vi "eventILCCommunication.vi"(8 "error in (no error)":errorcluster, 9 "TimeoutActuatorIds":i32[](array[numeric]), 10 "Timestamp":T1, 11 "Publisher in":refnum<class "Publisher.lvclass">) -> (0 "error out":errorcluster, 3 "Publisher out":refnum<class "Publisher.lvclass">)   [LabVIEW 2016, in "Publisher.lvclass"]
uses:
  Publisher.lvclass
  DataTypes/Topics/Parts/Timestamp.ctl
  Publisher.lvclass/Publisher.ctl
  DataTypes/Topics/EventILCCommunication.ctl
  Communicator/M1M3SAL/M1M3SAL.lvclass/M1M3SAL.ctl
  Communicator/M1M3SAL/writeHeader.vi
  Communicator/M1M3SAL/writeDBL.vi
  Communicator/M1M3SAL/writeI32.vi
  Communicator/M1M3SAL/writeBoolean.vi
  Communicator/M1M3SAL/writeU8.vi
  DataTypes/Topics/M1M3SupportTopics.lvlib
  Communicator/M1M3SAL/M1M3SAL.lvclass
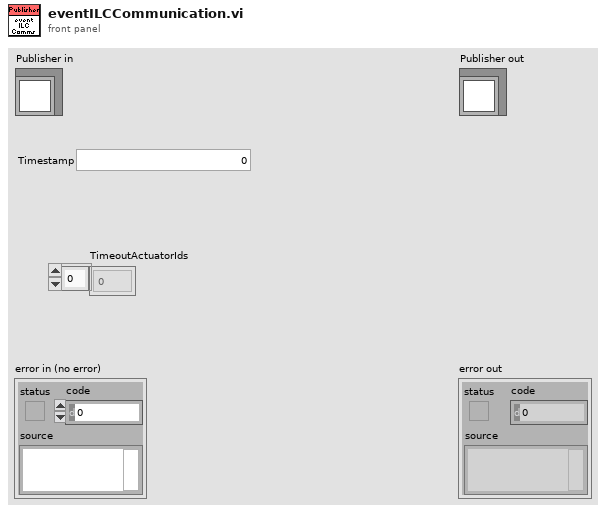
[diagram p1: front panel]
types:
  T1 = typedef "M1M3SupportTopics.lvlib/Timestamp.ctl" = dbl
  T2 = typedef "M1M3SupportTopics.lvlib/EventILCCommunication.ctl" = cluster{"Timestamp":T1, "ActuatorId":i32, "CommunicationOK":bool}
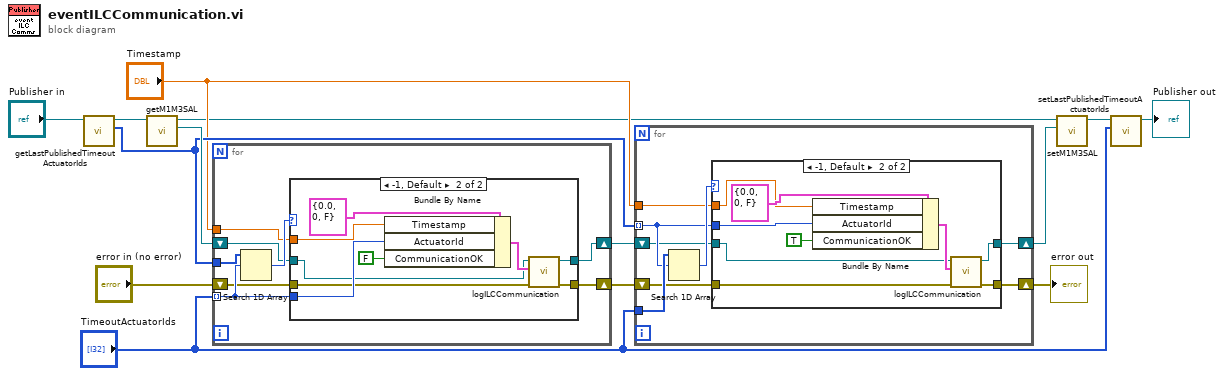
[diagram p0: block diagram]
diagram:
  n1 = call "getLastPublishedTimeoutActuatorIds.vi"("Publisher in"="Publisher in") -> ("LastPublishedTimeoutActuatorIds"=w11:i32[], "Publisher out"=w13:refnum<class "Publisher.lvclass">)  [unwired: 9 in]
  n2 = call "getM1M3SAL.vi"("Publisher in"=w13) -> ("M1M3SAL"=w12:refnum<class "M1M3SAL.lvclass">, "Publisher out"=w6:refnum<class "Publisher.lvclass">)  [unwired: 9 in]
  n3 = for {
    tunnel: "TimeoutActuatorIds" -> [w20] mode=indexing
    tunnel: w11 -> [w22]
    tunnel: "Timestamp" -> [w19]
    shift-right: [w17] -> w1
    shift-left: w12 -> [w18]
    shift-right: [w15] -> w3
    shift-left: "error in (no error)" -> [w16]
    n4 = Search 1D Array(1D array=w22, element=w20) -> (index of element=w21:i32)  [unwired: 1 in]
    n5 = case shown="-1, Default" w21 {
      tunnel: w20 -> [_ w31]
      tunnel: w19 -> [_ w30]
      tunnel: w18 -> [w24 w28]
      tunnel: [w24 w27] -> w17
      tunnel: w16 -> [w23 w26]
      tunnel: [w23 w25] -> w15
      frame 0 {
      }
      frame -1, Default {
        n6 = Bundle By Name(cluster=T2 {"Timestamp"=0.0, "ActuatorId"=0, "CommunicationOK"=FALSE} ("EventILCCommunication"), "Timestamp"=w30, "ActuatorId"=w31, "CommunicationOK"=FALSE) -> (w29:T2)
        n7 = call "logILCCommunication.vi"("error in (no error)"=w26, "EventILCCommunication"=w29, "M1M3SAL in"=w28) -> ("error out"=w25:errorcluster, "M1M3SAL out"=w27:refnum<class "M1M3SAL.lvclass">)  [unwired: 7 in]
      }
    }
  }
  n8 = for {
    tunnel: w11 -> [w39] mode=indexing
    tunnel: "TimeoutActuatorIds" -> [w41]
    tunnel: "Timestamp" -> [w38]
    shift-right: [w36] -> w5
    shift-left: w1 -> [w37]
    shift-right: [w34] -> w2
    shift-left: w3 -> [w35]
    n9 = Search 1D Array(1D array=w41, element=w39) -> (index of element=w40:i32)  [unwired: 1 in]
    n10 = case shown="-1, Default" w40 {
      tunnel: w39 -> [_ w50]
      tunnel: w38 -> [_ w49]
      tunnel: w37 -> [w43 w47]
      tunnel: [w43 w46] -> w36
      tunnel: w35 -> [w42 w45]
      tunnel: [w42 w44] -> w34
      frame 0 {
      }
      frame -1, Default {
        n11 = Bundle By Name(cluster=T2 {"Timestamp"=0.0, "ActuatorId"=0, "CommunicationOK"=FALSE} ("EventILCCommunication"), "Timestamp"=w49, "ActuatorId"=w50, "CommunicationOK"=TRUE) -> (w48:T2)
        n12 = call "logILCCommunication.vi"("error in (no error)"=w45, "EventILCCommunication"=w48, "M1M3SAL in"=w47) -> ("error out"=w44:errorcluster, "M1M3SAL out"=w46:refnum<class "M1M3SAL.lvclass">)  [unwired: 7 in]
      }
    }
  }
  "error out" <- w2
  n13 = call "setM1M3SAL.vi"("M1M3SAL"=w5, "Publisher in"=w6) -> ("Publisher out"=w8:refnum<class "Publisher.lvclass">)  [unwired: 9 in]
  n14 = call "setLastPublishedTimeoutActuatorIds.vi"("LastPublishedTimeoutActuatorIds"="TimeoutActuatorIds", "Publisher in"=w8) -> ("Publisher out"=→"Publisher out":refnum<class "Publisher.lvclass">)  [unwired: 9 in]
